vi "get_inputs.vi"() -> (3 "Inputs":T1)   [LabVIEW 2013]
uses:
  joystick_vals.ctl
  <vilib>/Rock Robotics/WPI/Joystick/WPI_JoystickButtonState.ctl
  inputs.ctl
  drive/drive_inputs.ctl
  flinger/flinger_inputs.ctl
  <vilib>/Rock Robotics/WPI/Joystick/WPI_JoystickGetSetRefNum.vi
panel:
  in  "Inputs 2":T1
  in  "Joysticks 2":T4
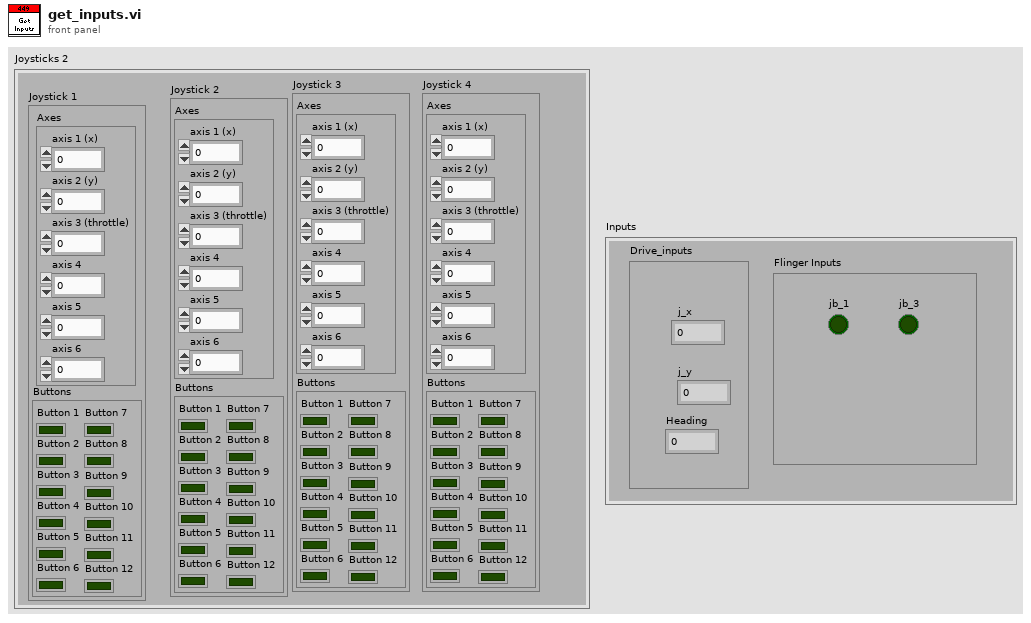
[diagram p1: front panel]
types:
  T1 = typedef "inputs.ctl" = cluster{"Drive_inputs":T2, "Flinger Inputs":T3}
  T2 = typedef "drive_inputs.ctl" = cluster{"j_x":dbl, "j_y":dbl, "Heading":dbl}
  T3 = typedef "flinger_inputs.ctl" = cluster{"jb_1":bool, "jb_3":bool}
  T4 = typedef "joystick_vals.ctl" = cluster{"Joystick 1":cluster{"Axes":cluster{"axis 1 (x)":dbl, "axis 2 (y)":dbl, "axis 3 (throttle)":dbl, "axis 4":dbl, "axis 5":dbl, "axis 6":dbl}, "Buttons":T5}, "Joystick 2":cluster{"Axes":cluster{"axis 1 (x)":dbl, "axis 2 (y)":dbl, "axis 3 (throttle)":dbl, "axis 4":dbl, "axis 5":dbl, "axis 6":dbl}, "Buttons":T5}, "Joystick 3":cluster{"Axes":cluster{"axis 1 (x)":dbl, "axis 2 (y)":dbl, "axis 3 (throttle)":dbl, "axis 4":dbl, "axis 5":dbl, "axis 6":dbl}, "Buttons":T5}, "Joystick 4":cluster{"Axes":cluster{"axis 1 (x)":dbl, "axis 2 (y)":dbl, "axis 3 (throttle)":dbl, "axis 4":dbl, "axis 5":dbl, "axis 6":dbl}, "Buttons":T5}}
  T5 = typedef "WPI_JoystickButtonState.ctl" = cluster{"Button 1":bool, "Button 2":bool, "Button 3":bool, "Button 4":bool, "Button 5":bool, "Button 6":bool, "Button 7":bool, "Button 8":bool, "Button 9":bool, "Button 10":bool, "Button 11":bool, "Button 12":bool}
  T6 = typedef "WPI_JoystickDevRef.ctl" = cluster{"Device":T7}
  T7 = typedef "WPI_JoystickDeviceEnum.ctl" = enum16{"USB 1", "USB 2", "USB 3", "USB 4", "Kinect 1", "Kinect 2"}
  T8 = cluster{"axis 1 (x)":dbl, "axis 2 (y)":dbl, "axis 3 (throttle)":dbl, "axis 4":dbl, "axis 5":dbl, "axis 6":dbl}
  T9 = cluster{"Axes":cluster{"axis 1 (x)":dbl, "axis 2 (y)":dbl, "axis 3 (throttle)":dbl, "axis 4":dbl, "axis 5":dbl, "axis 6":dbl}, "Buttons":T5}
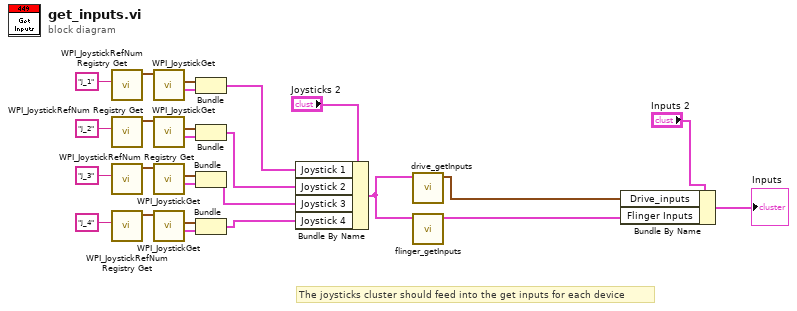
[diagram p0: block diagram]
diagram:
  # "The joysticks cluster should feed into the get inputs for each device"
  n1 = call <vilib>:"WPI_JoystickRefNum Registry Get.vi"("refnum name"="j_1") -> ("JoystickDevRef"=w21:T6)  [unwired: 9 in, 1 out]
  n2 = call <vilib>:"WPI_JoystickRefNum Registry Get.vi"("refnum name"="j_2") -> ("JoystickDevRef"=w17:T6)  [unwired: 9 in, 1 out]
  n3 = call <vilib>:"WPI_JoystickRefNum Registry Get.vi"("refnum name"="j_3") -> ("JoystickDevRef"=w13:T6)  [unwired: 9 in, 1 out]
  n4 = call <vilib>:"WPI_JoystickRefNum Registry Get.vi"("refnum name"="j_4") -> ("JoystickDevRef"=w25:T6)  [unwired: 9 in, 1 out]
  n5 = call <vilib>:"WPI_JoystickGet.vi"("JoystickDevRef"=w21) -> ("Buttons"=w20:T5, "Axes"=w19:T8)  [unwired: 4 in, 1 out]
  n6 = call <vilib>:"WPI_JoystickGet.vi"("JoystickDevRef"=w17) -> ("Buttons"=w16:T5, "Axes"=w15:T8)  [unwired: 4 in, 1 out]
  n7 = call <vilib>:"WPI_JoystickGet.vi"("JoystickDevRef"=w13) -> ("Buttons"=w12:T5, "Axes"=w11:T8)  [unwired: 4 in, 1 out]
  n8 = call <vilib>:"WPI_JoystickGet.vi"("JoystickDevRef"=w25) -> ("Buttons"=w24:T5, "Axes"=w23:T8)  [unwired: 4 in, 1 out]
  n9 = Bundle("Axes"=w19, "Buttons"=w20) -> (w9:T9)  [unwired: 1 in]
  n10 = Bundle("Axes"=w15, "Buttons"=w16) -> (w8:T9)  [unwired: 1 in]
  n11 = Bundle("Axes"=w11, "Buttons"=w12) -> (w7:T9)  [unwired: 1 in]
  n12 = Bundle("Axes"=w23, "Buttons"=w24) -> (w6:T9)  [unwired: 1 in]
  n13 = Bundle By Name(cluster="Joysticks 2", "Joystick 1"=w9, "Joystick 2"=w8, "Joystick 3"=w7, "Joystick 4"=w6) -> (w2:T4)
  n14 = call "drive_getInputs.vi"("Joysticks"=w2) -> ("Drive"=w3:T2)  [unwired: 10 in]
  n15 = call "flinger_getInputs.vi"("Joysticks"=w2) -> ("Flinger Inputs"=w1:T3)  [unwired: 10 in]
  n16 = Bundle By Name(cluster="Inputs 2", "Drive_inputs"=w3, "Flinger Inputs"=w1) -> (→"Inputs":T1)
